vi "Robot Global Data.vi"() -> ()   [LabVIEW 2019]
doc: "This global VI can contain as many global variables as you need. Place a control on the panel, give it a good name. To read or write to it from a VI, drag the icon to the diagram of that VI. You can also drag from the project. Click on the node to change which global you access. You shouldn't have multiple locations writing to a global or it will cause a race-condition."
uses:
  <vilib>/Rock Robotics/WPI/Camera/WPI_CameraImageSize.ctl
  <vilib>/Rock Robotics/WPI/DriverStation/WPI_DriverStationRobotMode2.ctl
panel:
  out "FINISH":bool
  in  "Right Drive Max Output":dbl=1.0 min=-1.0 max=1.0 step=0.01
  in  "Right Drive Min Output":dbl=-1.0 min=-1.0 max=1.0 step=0.01
  in  "Right Drive I Zone":dbl step=0.01
  in  "Right Drive F Gain":dbl step=0.01
  in  "Right Drive D Gain":dbl step=0.01
  in  "Right Drive I Gain":dbl step=0.01
  in  "Right Drive P Gain":dbl min=0.0 step=0.01
  in  "Right Drive Applied Output":dbl
  in  "Right Drive Velocity Setpoint":dbl
  in  "Right Drive Distance":dbl
  in  "Right Drive Velocity":dbl
  in  "Left Drive Applied Output":dbl
  in  "Left Drive Max Output":dbl=1.0 min=-1.0 max=1.0 step=0.01
  in  "Left Drive Min Output":dbl=-1.0 min=-1.0 max=1.0 step=0.01
  in  "Left Drive I Zone":dbl step=0.01
  in  "Left Drive F Gain":dbl step=0.01
  in  "Left Drive D Gain":dbl step=0.01
  in  "Left Drive I Gain":dbl step=0.01
  in  "Left Drive P Gain":dbl min=0.0 step=0.01
  in  "Left Drive Velocity Setpoint":dbl
  in  "Left Drive Distance":dbl
  in  "Left Drive Velocity":dbl
  in  "Robot Mode":T1
  in  "image size":T2=enum."320x240"
  in  "Enable Vision":bool
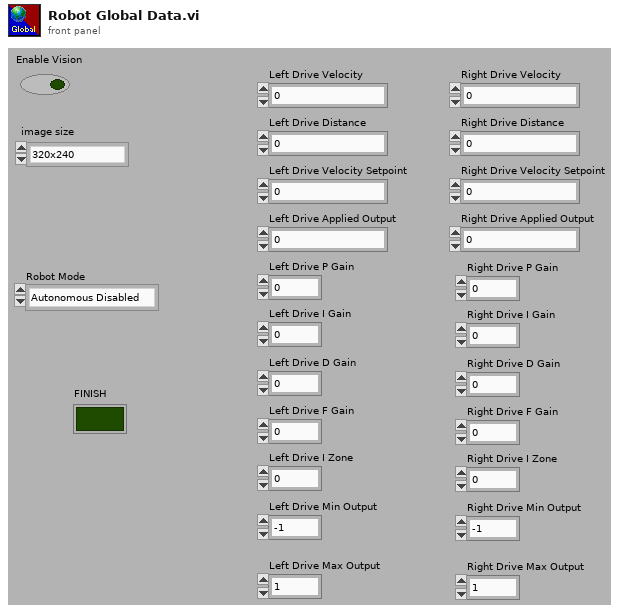
[diagram p1: front panel]
types:
  T1 = typedef "WPI_DriverStationRobotMode2.ctl" = enum16{"Autonomous Disabled", "Autonomous Enabled", "Teleop Disabled", "Teleop Enabled", "Disconnected", "Finish", "Test Disabled", "Test Enabled", "Emergency Stopped"}
  T2 = typedef "WPI_CameraImageSize.ctl" = enum16{"640x480", "320x240", "160x120", "Custom"}
diagram:
